vi "Test Kinematics.vi"() -> ()   [LabVIEW 2013]
uses:
  <vilib>/Analysis/Matrix/Datatypes/RealMatrix.ctl
  SubVIs/SR6-NC Arm/SR6-NC Arm.lvclass
  <vilib>/robotics/Kinematics/Robot/Forward Kinematics (Point).vi
  <vilib>/robotics/Kinematics/NI_Kinematics.lvlib
  <vilib>/robotics/Kinematics/Plotting/NI_Robotics_3DKinematics.lvlib
  <vilib>/Analysis/Matrix/NI_Matrix.lvlib
panel:
  out "end effector transform 2":dbl[][][](array[numeric])
  out "joint positions":T1
  out "end effector transform":T1
  in  "stop":bool
  out "3D Picture":refnum<vi>(3d-picture)
  in  "Joints":dbl[](array[slide])=[0.0, 0.0, 0.0, 0.0, 0.0, -3.673469387755098] scale=-180.0..180.0
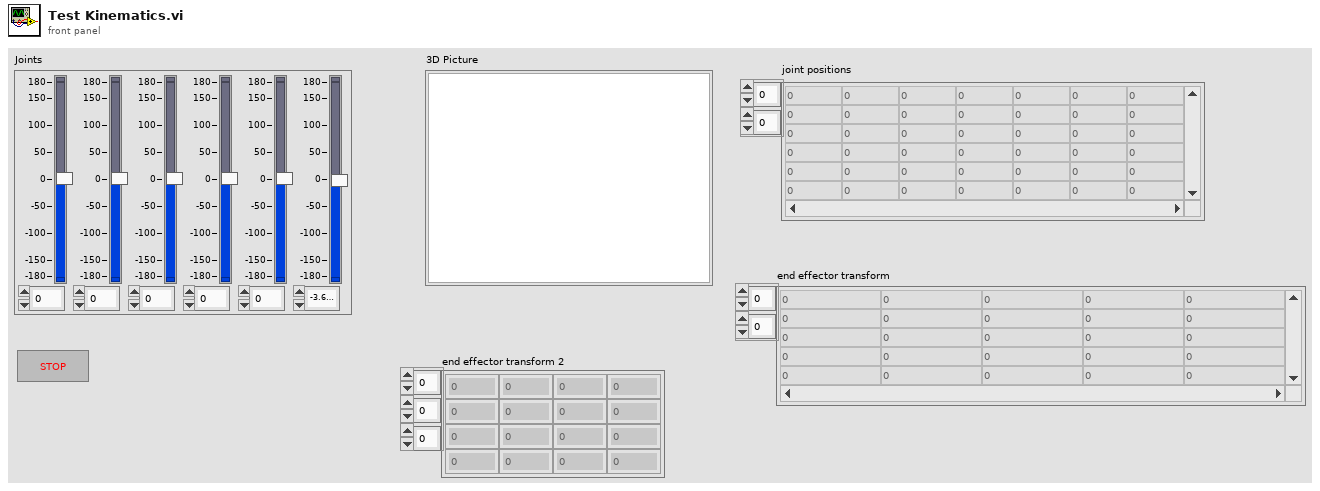
[diagram p1: front panel]
types:
  T1 = typedef "NI_Matrix.lvlib/RealMatrix.ctl" = dbl[][]
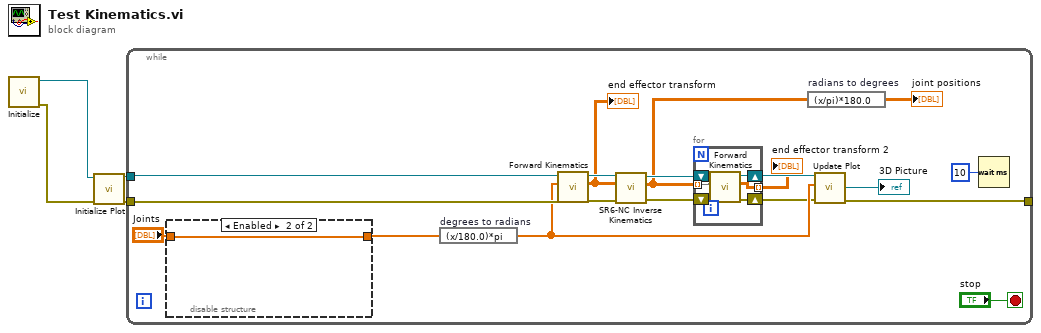
[diagram p0: block diagram]
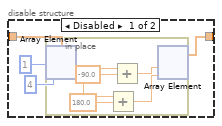
[diagram p2: hidden frame]
diagram:
  n1 = call "Initialize.vi"() -> ("error out"=w1:errorcluster, "SR6-NC Arm out"=w4:refnum<class "SR6-NC Arm.lvclass">)  [unwired: 10 in]
  n2 = call <vilib>:"Initialize Plot.vi"("error in (no error)"=w1, "serial arm in"=w4) -> ("error out"=w2:errorcluster, "serial arm out"=w3:refnum<class "SR6-NC Arm.lvclass">)  [unwired: 8 in]
  n3 = while {
    tunnel: w3 -> [w19]
    tunnel: w2 -> [w18]
    tunnel: [w21] -> _
    stop <- "stop" stop-if-true
    n4 = disable-structure shown="Enabled" {
      disable-tunnel: "Joints" -> [w33 w40]
      disable-tunnel: [w31 w40] -> w11
      frame Disabled {
        n5 = in-place {
          n6 = in-place-array #1(w33, 1, 4) -> (w39:dbl, w36:dbl)
          n7 = Add(x=w36, y=180.0) -> (x+y=w34:dbl)
          n8 = Add(x=w39, y=-90.0) -> (x+y=w37:dbl)
          n9 = in-place-array #1(w37, w34) -> (w31:dbl[])  [unwired: 2 out]
        }
      }
      frame Enabled {
      }
    }
    n10 = expression code="(x/180.0)*pi" "degrees to radians"(w11) -> (w17:dbl[])
    n11 = call-poly <vilib>:"Forward Kinematics.vi"("error in (no error)"=w18, "joint positions"=w17, "serial arm in"=w19) -> ("error out"=w16:errorcluster, "end effector transform"=w14:T1, "serial arm out"=w15:refnum<class "SR6-NC Arm.lvclass">)  [unwired: 6 in]
    "end effector transform" <- w14
    n12 = call-dynamic "SR6-NC Inverse Kinematics.vi"("error in (no error)"=w16, "end effector transform"=w14, "SR6-NC Arm in"=w15) -> ("error out"=w8:errorcluster, "joint positions"=w6:T1, "SR6-NC Arm out"=w10:refnum<class "SR6-NC Arm.lvclass">)  [unwired: 5 in, 1 out]
    n13 = for {
      shift-right: [w28] -> w9
      shift-left: w10 -> [w29]
      shift-right: [w26] -> w7
      shift-left: w8 -> [w27]
      tunnel: w6 -> [w25] mode=indexing
      tunnel: [w24] -> w5 mode=indexing
      n14 = call-poly <vilib>:"Forward Kinematics.vi"("error in (no error)"=w27, "joint positions"=w25, "serial arm in"=w29) -> ("error out"=w26:errorcluster, "end effector transform"=w24:T1, "serial arm out"=w28:refnum<class "SR6-NC Arm.lvclass">)  [unwired: 6 in]
    }
    "end effector transform 2" <- w5
    n15 = expression code="(x/pi)*180.0" "radians to degrees"(w6) -> (→"joint positions":T1)
    n16 = call <vilib>:"Update Plot.vi"("error in (no error)"=w7, "joint positions"=w17, "serial arm in"=w9) -> ("error out"=w21:errorcluster, "serial arm scene"=→"3D Picture":refnum<vi>)  [unwired: 6 in, 1 out]
    n17 = Wait (ms)(milliseconds to wait=u32 10) -> ()  [unwired: 1 out]
  }
